vi "Lifter_create_file To Network.vi"(8 "error in (no error)":errorcluster, 11 "File Name":string) -> (0 "error out":errorcluster, 3 "dup path":path)   [LabVIEW 2019]
panel:
  out "concatenated string":string
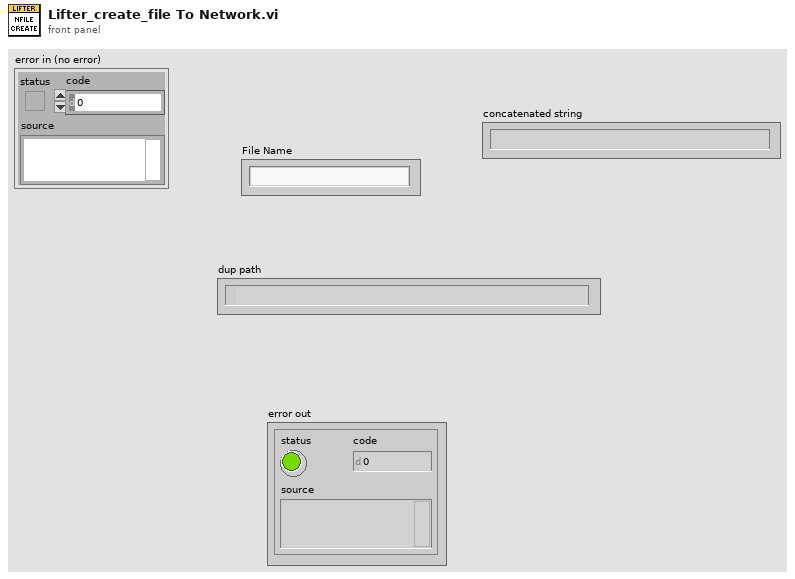
[diagram p1: front panel]
types:
  T1 = enum16{"open", "replace", "create", "open or create", "replace or create", "replace or create with confirmation"}
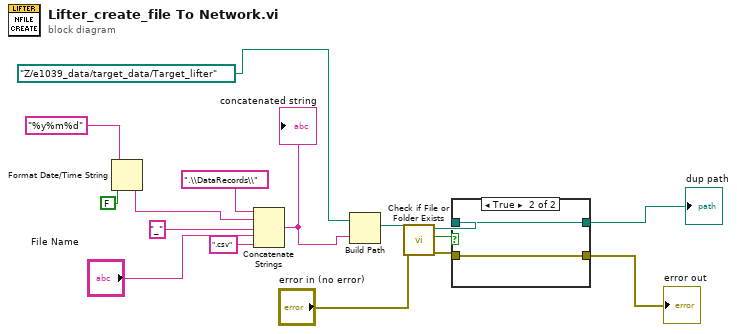
[diagram p0: block diagram]
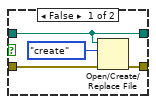
[diagram p2: hidden frame]
diagram:
  n1 = Format Date/Time String(time format string (%c)="%y%m%d", UTC format=FALSE) -> (date/time string=w9:string)  [unwired: 1 in]
  n2 = Concatenate Strings(".\\DataRecords\\" ("string"), w9, "_" ("string"), "File Name", ".csv" ("string")) -> (w16:string)
  "concatenated string" <- w16
  n3 = Build Path(base path=path "Z:/e1039_data/target_data/Target_lifter" ("path"), name or relative path=w16) -> (appended path=w15:path)
  n4 = call <vilib>:"Check if File or Folder Exists.vi"("error in (no error)"="error in (no error)", "path"=w15) -> ("error out"=w13:errorcluster, "file or folder exists?"=w12:bool, "dup path"=w14:path)  [unwired: 7 in]
  n5 = case shown="True" w12 {
    tunnel: w14 -> [w18 w21]
    tunnel: [w19 w22] -> w6
    tunnel: [w18 w21] -> w7
    tunnel: w13 -> [w17 w22]
    frame False {
      n6 = Open/Create/Replace File(file path (use dialog)=w18, error in=w17, operation (0:open)=T1."create") -> (error out=w19:errorcluster)  [unwired: 3 in, 2 out]
    }
    frame True {
    }
  }
  "dup path" <- w7
  "error out" <- w6
